vi "ANN on Simulated Starter Kit 1.0.vi"() -> ()   [LabVIEW 2017]
doc: "This VI demonstrates how to descontrol a simulated Starter Kit robot based on an Artificial Neural Network (ANN) algorithm. \n\nThe Starter Kit robot will track the path of red dots at the <b>Linear Velocity</b> you specify."
uses:
  ANN/ModelType.ctl
  ANN/ESN network/ESN_Network.ctl
  <vilib>/Analysis/Matrix/Datatypes/RealMatrix.ctl
  ANN/Trajectory.ctl
  <vilib>/robotics/Simulator/Engine/ctl/DeviceID.ctl
  <vilib>/Platform/TimedLoop/XDataNode/timing_clust.ctl
  <vilib>/Platform/TimedLoop/XDataNode/nitl_modes.ctl
  <vilib>/Platform/TimedLoop/XDataNode/wakeup.ctl
  ANN/ESN network/UserSettingsESN.ctl
  <vilib>/robotics/Simulator/Interface/Simulator References/Get Robot Body Reference.vi
  <vilib>/robotics/Simulator/Interface/Simulator References/Get World Reference.vi
  <instrlib>/DC Motor Controller/HAIOL/DC Motor Controller.lvclass
  <vilib>/Platform/TimedLoop/XDataNode/XDataNode.xnode
  <vilib>/robotics/Simulator/NI_Robotics_Simulator.lvlib
  <vilib>/Platform/TimedLoop/XDataNode/XDNodeRunTimeDep.lvlib
  <instrlib>/DC Motor Controller/HAIOL/Simulator/DC Motor Controller Simulator.lvclass
  <vilib>/Analysis/Matrix/NI_Matrix.lvlib
  <vilib>/gmath/NI_Gmath.lvlib
  <resource>/objmgr/LVODE.rc
panel:
  out "ESN trained 2":T1
  in  "Render Destination":enum16{"Scene Window", "Scene Display"}(ring)=enum."Scene Display"
  out "Location Error":cluster{"x":dbl, "y":dbl, "Orientation":dbl}(graph)
  out "Motor":dbl[][](graph)
  out "MSE":dbl
  in  "Linear Velocity":dbl=0.5 min=0.0 max=1.0 step=0.01
  in  "Model Type":T3=1 items=["Analytical Kinematic Model", "ANN Kinematic Model"]
  in  "Quit":bool
  out "Waveform WR_WL":dbl[][](graph)
  out "Time of Acquisition":i64
  out "Waveform V_W":dbl[][](graph)
  out "V_W":dbl[][](array[numeric])
  out "WR_WL":dbl[][](array[numeric])
  out "Data_WorkSpace":dbl[][](array[numeric])
  out "Percentage":string
  out "Data Acquisition Progress":dbl(slide) scale=0.0..100.0
  in  "WayPoints":cluster{sgl, sgl}[](array[cluster])=[{0.5, 0.5}, {0.5, 1.0}, {0.5, 1.5}, {0.5, 2.0}, {0.5, 2.5}, {0.5, 3.0}, {0.79999995, 3.4}, {1.2, 3.7}, {1.7, 3.7}, {2.1, 4.0}, {2.4, 4.4}, {2.7, 4.8}, {3.0, 5.2}, {3.4, 5.5}, {3.9, 5.5}, {4.4, 5.5}, {4.8, 5.8}, {5.3, 5.8}, {5.85, 5.5}, {5.85, 5.0}, {5.85, 4.5}, {5.4, 4.1}, {5.0, 3.8}, {4.7, 3.4}, {4.4, 3.0}, {4.1, 2.6}, {3.8, 2.2}, {3.8, 1.7}, {3.8, 1.2}, {4.1, 0.79999995}, {4.5, 0.5}, {5.0, 0.5}, {5.4, 0.79999995}]
  in  "method":i32(ring)=3 items=["nearest", "linear", "spline", "cubic Hermite"]
  in  "ntimes":i32=5
  out "trajectory":T4
  out "Path Graph":cluster{"yi":dbl[], "yi":dbl[]}[](graph)
  in  "Next":bool
  out "data acquisition status":bool
  in  "ESN trained":T1={"output to internal feedback?"=FALSE, "output to output feedback?"=FALSE, "input to output feedforward?"=TRUE, "number of input (K)"=2, "number of internal (N)"=222, "number of output (L)"=2, "input normalization vector"=[0.6006126900000001, 2.94100566], "output restore vector"=[30.199380389999998, 30.418265820000002], "input weight (N*K)"=array222x2[444 elements], "feedback weight (N*L)"=[], "internal weight (N*N)"=array222x222[49284 elements], "output weight (L*(K+N+L))"=array2x224[448 elements]}
  out "back status":bool
  out "3D Picture":refnum<vi>(3d-picture)
  # "Path Determintion"
  # "ANN Training"
  # "Mean\nSquare\nError"
  # "the range [0,1]."
  # "V,  W,  WL,  WR"
  # "Workspace Calculations"
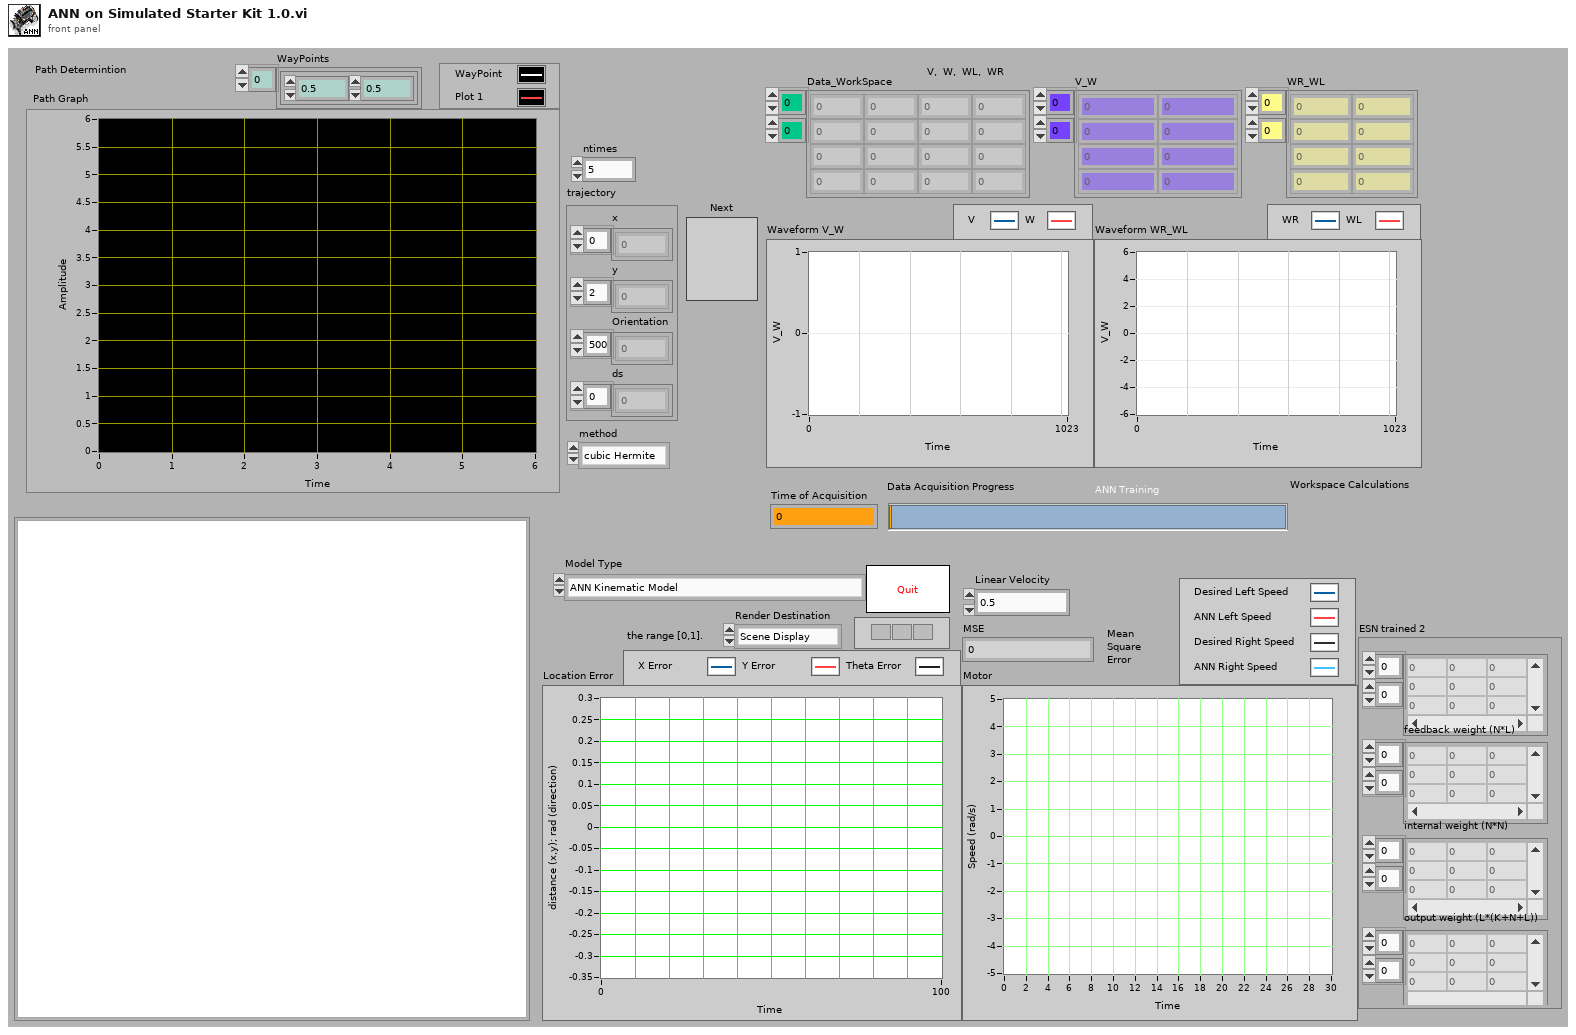
[diagram p1: front panel]
types:
  T1 = typedef "ESN_Network.ctl" = cluster{"output to internal feedback?":bool, "output to output feedback?":bool, "input to output feedforward?":bool, "number of input (K)":i32, "number of internal (N)":i32, "number of output (L)":i32, "input normalization vector":dbl[], "output restore vector":dbl[], "input weight (N*K)":T2, "feedback weight (N*L)":T2, "internal weight (N*N)":T2, "output weight (L*(K+N+L))":T2}
  T2 = typedef "NI_Matrix.lvlib/RealMatrix.ctl" = dbl[][]
  T3 = typedef "ModelType.ctl" = u16
  T4 = typedef "Trajectory.ctl" = cluster{"x":dbl[], "y":dbl[], "Orientation":dbl[], "ds":dbl[]}
  T5 = typedef "NI_Robotics_Simulator.lvlib/DeviceID.ctl" = cluster{"robot ID":string, "sensor/actuator ID":string}
  T6 = typedef "XDNodeRunTimeDep.lvlib/timing_clust.ctl" = cluster{"Expected End [f-1]":u64, "Actual End [f-1]":u64, "Finished Late? [f-1]":bool, "Expected End [i-1]":u64, "Actual End [i-1]":u64, "Finished Late? [i-1]":bool, "Expected Start [i]":u64, "Actual Start [i]":u64, "Expected Start [f]":u64, "Actual Start [f]":u64, "Source Name":string, "Structure Name":string, "Period":i64, "Deadline":i64, "Offset":i64, "Start":i64, "Priority":i32, "Timeout":i32, "Mode":T7, "Wakeup Reason":T8, "Error":errorcluster, "Source Type":string, "Secondary Source Type":string, "Global End Time":u64, "Global Start Time":u64, "Frame Duration":u64, "Iteration Duration":u64, "Assigned CPU":i32, "I/O Scan Engine Mode":u32}
  T7 = typedef "XDNodeRunTimeDep.lvlib/nitl_modes.ctl" = enum32{"No Change", "Process missed periods, maintain original phase", "Discard missed periods, maintain original phase", "Process missed periods, ignore original phase", "Discard missed periods, ignore original phase"}
  T8 = typedef "XDNodeRunTimeDep.lvlib/wakeup.ctl" = enum32{"Normal", "Aborted", "Asynchronous wakeup", "Timing source error", "Timed loop error", "Timeout"}
  T9 = typedef "UserSettingsESN.ctl" = cluster{"output to internal feedback?":bool, "output to output feedback?":bool, " input to output feedforward?":bool, "number of input (K)":i32, "number of internal (N)":i32, "number of output (L)":i32}
  T10 = typedef "VehiclePosture.ctl" = cluster{"x":dbl, "y":dbl, "Orientation":dbl}
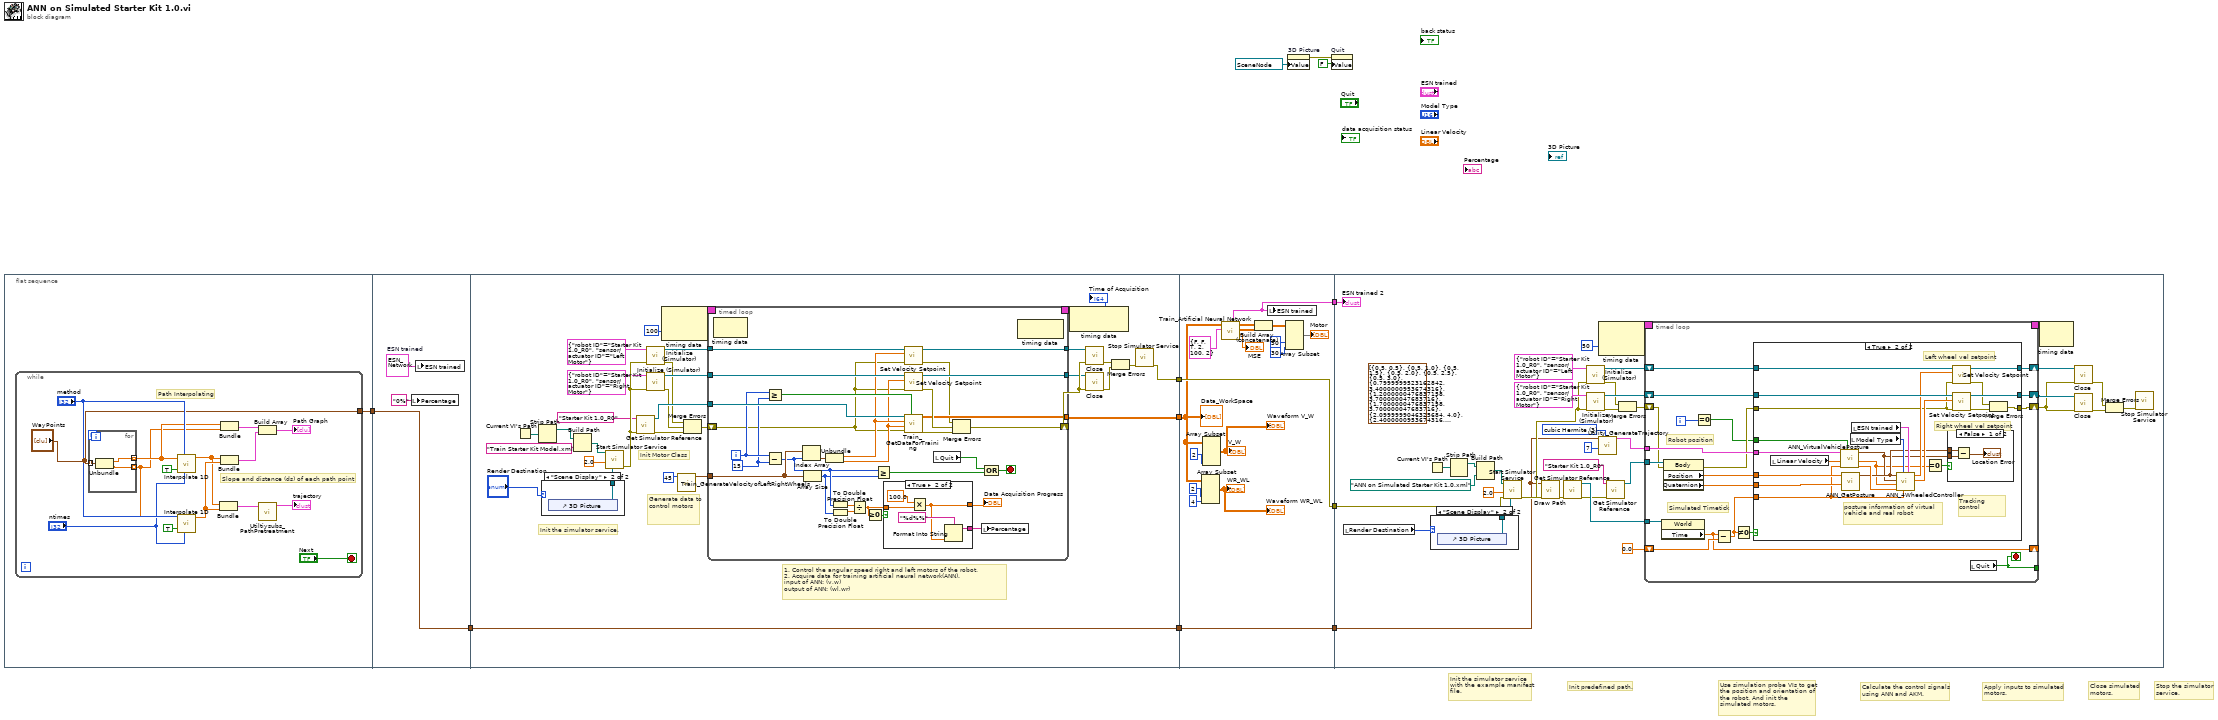
[diagram p0: block diagram]
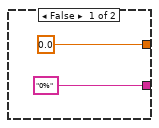
[diagram p2: hidden frame]
diagram:
  # "Init the simulator service\nwith the example manifest\nfile."
  # "Stop the simulator\nservice."
  # "Close simulated\nmotors."
  # "Apply inputs to simulated\nmotors."
  # "Calculate the control signals\nusing ANN and AKM."
  # "Use simulation probe VIs to get\nthe position and orientation of\nthe robot. And init the\nsimulated motors."
  # "Init predefined path."
  n1 = flat-sequence {
    tunnel: [w12] -> w6
    tunnel: w6 -> [w31]
    tunnel: [w31] -> w5
    tunnel: [w38] -> w7
    tunnel: w5 -> [w38]
    tunnel: [w37] -> w3
    tunnel: [w35] -> w2
    tunnel: [w119] -> w8
    tunnel: w7 -> [w119]
    tunnel: [w118] -> w4
    tunnel: w3 -> [w118]
    tunnel: w2 -> [w117]
    tunnel: [w111] -> w1
    tunnel: w8 -> [w130]
    tunnel: w4 -> [w131]
    tunnel: w1 -> [w128]
    frame #0 {
      n2 = while {
        tunnel: ["WayPoints"] -> w12
        stop <- "Next" stop-if-true
        # "Slope and distance (ds) of each path point"
        # "Path Interpolating"
        n3 = for {
          tunnel: "WayPoints" -> [w30] mode=indexing
          tunnel: [w29] -> w19 mode=indexing
          tunnel: [w28] -> w13 mode=indexing
          n4 = Unbundle(w30) -> (w29:sgl, w28:sgl)
        }
        n5 = call <vilib>:"Interpolate 1D.vi"("ntimes"="ntimes", "method"="method", "X is monotonic"=TRUE, "Y"=w19) -> ("yi"=w22:dbl[])  [unwired: 5 in, 2 out]
        n6 = call <vilib>:"Interpolate 1D.vi"("ntimes"="ntimes", "method"="method", "X is monotonic"=TRUE, "Y"=w13) -> ("yi"=w23:dbl[])  [unwired: 5 in, 2 out]
        n7 = Bundle("yi"=w22, "yi"=w23) -> (w24:cluster{"yi":dbl[], "yi":dbl[]})  [unwired: 1 in]
        n8 = Bundle("yi"=w22, "yi"=w23) -> (w20:cluster{"yi":dbl[], "yi":dbl[]})  [unwired: 1 in]
        n9 = Bundle(w19, w13) -> (w14:cluster{sgl[], sgl[]})  [unwired: 1 in]
        n10 = Build Array(w14, w20) -> (→"Path Graph":cluster{"yi":dbl[], "yi":dbl[]}[])
        n11 = call "Utiltiysubs_PathPretreatment.vi"("original trajectory"=w24) -> ("trajectory"=→"trajectory":T4)  [unwired: 10 in]
      }
    }
    frame #1 {
      w33 = T1 {"output to internal feedback?"=FALSE, "output to output feedback?"=FALSE, "input to output feedforward?"=TRUE, "number of input (K)"=2, "number of internal (N)"=222, "number of output (L)"=2, "input normalization vector"=[0.6006126900000001, 2.94100566], "output restore vector"=[30.199380389999998, 30.418265820000002], "input weight (N*K)"=array222x2[444 elements], "feedback weight (N*L)"=[], "internal weight (N*N)"=array222x222[49284 elements], "output weight (L*(K+N+L))"=array2x224[448 elements]}  # ESN trained
      n12 = local write "Percentage"("0%" ("Percentage")) -> ()
      n13 = local write "ESN trained"(w33) -> ()
    }
    frame #2 {
      # "1. Control the angular speed right and left motors of the robot.\n2. Acquire data for training artificial neural network(ANN).\ninput of ANN: (v,w)\noutput of ANN: (wl,wr)"
      # "Generate data to control motors"
      # "Init Motor Class"
      # "Init the simulator service."
      n14 = Current VI's Path() -> (path=w43:path)
      n15 = Strip Path(path=w43) -> (stripped path=w42:path)  [unwired: 1 out]
      n16 = case shown="\"Scene Display\"" "Render Destination" {
        tunnel: [_ w110] -> w40
        frame "Scene Window", Default {
        }
        frame "Scene Display" {
          n17 = control-ref of="3D Picture"() -> (w110:refnum<vi>)
        }
      }
      n18 = Build Path(base path=w42, name or relative path="Train Starter Kit Model.xml" ("ManifestFile")) -> (appended path=w41:path)
      n19 = call <vilib>:"Start Simulator Service.vi"("3D picture refnum"=w40, "step size (ms)"=2.0 ("stepsize(ms)"), "manifest file"=w41) -> ("error out"=w60:errorcluster)  [unwired: 8 in]
      n20 = call-poly <vilib>:"Get Simulator Reference.vi"("error in (no error)"=w60, "robot ID"="Starter Kit 1.0_R0") -> ("error out"=w45:errorcluster, "robot body ref"=w56:refnum<k20>)  [unwired: 8 in]
      n21 = call <instrlib>:"Initialize (Simulator).vi"("error in (no error)"=w60, "Device ID"=T5 {"robot ID"="Starter Kit 1.0_R0", "sensor/actuator ID"="Left Motor"}) -> ("error out"=w48:errorcluster, "DC Motor Controller out"=w53:refnum<class "DC Motor Controller.lvclass">)  [unwired: 8 in]
      n22 = call <instrlib>:"Initialize (Simulator).vi"("error in (no error)"=w60, "Device ID"=T5 {"robot ID"="Starter Kit 1.0_R0", "sensor/actuator ID"="Right Motor"}) -> ("error out"=w47:errorcluster, "DC Motor Controller out"=w54:refnum<class "DC Motor Controller.lvclass">)  [unwired: 8 in]
      n23 = node-c288(i64 100 ("Period")) -> (w66:T6)  [unwired: 1 in]
      n24 = call "Train_GenerateVelocityofLeftRightWheels.vi"("samples"=45) -> ("speed of Left and Right Wheels (rad/s)"=w55:cluster{dbl, dbl}[])  [unwired: 10 in]
      n25 = Merge Errors(w48, w47, w45) -> (w52:errorcluster)
      n26 = timed-loop {
        shift-right: [w95] -> w61
        shift-left: w52 -> [w72]
        tunnel: w53 -> [w94]
        tunnel: w54 -> [w93]
        tunnel: [w92] -> w58
        tunnel: [w91] -> w59
        tunnel: w55 -> [w90]
        tunnel: w56 -> [w88]
        tunnel: [w76] -> w35
        timing: w66 -> [_]
        timing-out: [_] -> w65
        i -> [w87]
        stop <- w74 stop-if-true
        w86 = 15 ("y")
        n27 = node-c288() -> ()  [unwired: 1 in, 1 out]
        n28 = Greater Or Equal?(x=w87, y=w86) -> (x >= y?=w85:bool)
        n29 = Subtract(x=w87, y=w86) -> (x-y=w89:i32)
        n30 = Index Array(array=w90, index=w89) -> (element=w84:cluster{dbl, dbl})
        n31 = Array Size(array=w90) -> (size(s)=w81:i32)
        n32 = Unbundle(w84) -> (w83:dbl, w82:dbl)
        n33 = To Double Precision Float(number=w89) -> (double precision float=w79:dbl)
        n34 = To Double Precision Float(number=w81) -> (double precision float=w80:dbl)
        n35 = Divide(x=w79, y=w80) -> (x/y=w70:dbl)
        n36 = Greater Or Equal To 0?(x=w70) -> (x >= 0?=w69:bool)
        n37 = Greater Or Equal?(x=w89, y=w81) -> (x >= y?=w75:bool)
        n38 = case shown="True" w69 {
          tunnel: w70 -> [_ w102]
          tunnel: ["0%" w99] -> w68
          tunnel: [0.0 w98] -> w67
          frame False {
          }
          frame True {
            n39 = Multiply(x=100.0 ("y"), y=w102) -> (x*y=w98:dbl)
            n40 = Format Into String(format string="%d%%", w98) -> (resulting string=w99:string)  [unwired: 2 in, 1 out]
          }
        }
        "Data Acquisition Progress" <- w67
        n41 = call-dynamic "Set Velocity Setpoint.vi"("error in (no error)"=w72, "CCW Velocity (0 rad/s)"=w83, "DC Motor Controller in"=w94) -> ("error out"=w71:errorcluster, "DC Motor Controller out"=w92:refnum<class "DC Motor Controller.lvclass">)  [unwired: 7 in]
        n42 = call-dynamic "Set Velocity Setpoint.vi"("error in (no error)"=w72, "CCW Velocity (0 rad/s)"=w82, "DC Motor Controller in"=w93) -> ("error out"=w77:errorcluster, "DC Motor Controller out"=w91:refnum<class "DC Motor Controller.lvclass">)  [unwired: 7 in]
        n43 = call "Train_GetDataForTraining.vi"("DataIn"=w85, "error in (no error)"=w72, "WR"=w82, "Wl"=w83, "robot body ref"=w88) -> ("error out"=w78:errorcluster, "Data"=w76:dbl[][])  [unwired: 5 in]
        n44 = local read "Quit"() -> (w73:bool)
        n45 = Merge Errors(w71, w77, w78) -> (w95:errorcluster)
        n46 = local write "Percentage"(w68) -> ()
        n47 = Compound Arithmetic op=OR(w73, w75) -> (w74:bool)
        n48 = node-c288() -> ()  [unwired: 1 in, 1 out]
      }
      n49 = node-c288(w65) -> (→"Time of Acquisition":i64)
      n50 = call-dynamic "Close.vi"("error in (no error)"=w61, "DC Motor Controller in"=w58) -> ("error out"=w62:errorcluster)  [unwired: 9 in]
      n51 = call-dynamic "Close.vi"("error in (no error)"=w61, "DC Motor Controller in"=w59) -> ("error out"=w63:errorcluster)  [unwired: 9 in]
      n52 = Merge Errors(w62, w63) -> (w64:errorcluster)
      n53 = call <vilib>:"Stop Simulator Service.vi"("error in (no error)"=w64) -> ("error out"=w37:errorcluster)  [unwired: 10 in]
    }
    frame #3 {
      n54 = Array Subset(array=w117, index (col)=2 ("index"), length (col)=4 ("length")) -> (→"WR_WL" →"Waveform WR_WL":dbl[][])  [unwired: 2 in]
      n55 = Array Subset(array=w117, length (col)=2 ("length")) -> (→"V_W" →"Waveform V_W":dbl[][])  [unwired: 3 in]
      n56 = call "Train_Artificial Neural Network.vi"("UserSettingsESN"=T9 {"output to internal feedback?"=FALSE, "output to output feedback?"=FALSE, " input to output feedforward?"=TRUE, "number of input (K)"=2, "number of internal (N)"=100, "number of output (L)"=2}, "Data"=w117) -> ("MSE"=→"MSE":dbl, "Wr"=w125:dbl[][], "Wl"=w126:dbl[][], "ESN trained"=w111:T1)  [unwired: 5 in, 1 out]
      n57 = Build Array (concatenate)(w126, w125) -> (w124:dbl[][])
      n58 = local write "ESN trained"(w111) -> ()
      n59 = Array Subset(array=w124, index (col)=50 ("index"), length (col)=30 ("length")) -> (→"Motor":dbl[][])  [unwired: 2 in]
      "Data_WorkSpace" <- w117
    }
    frame #4 {
      (unwired) cluster{sgl, sgl}[] [{0.5, 0.5}, {0.5, 1.0}, {0.5, 1.5}, {0.5, 2.0}, {0.5, 2.5}, {0.5, 3.0}, {0.79999995, 3.4}, {1.2, 3.7}, {1.7, 3.7}, {2.1, 4.0}, {2.4, 4.4}, {2.7, 4.8}, {3.0, 5.2}, {3.4, 5.5}, {3.9, 5.5}, {4.4, 5.5}, {4.8, 5.8}, {5.3, 5.8}, {5.85, 5.5}, {5.85, 5.0}, {5.85, 4.5}, {5.4, 4.1}, {5.0, 3.8}, {4.7, 3.4}, {4.4, 3.0}, {4.1, 2.6}, {3.8, 2.2}, {3.8, 1.7}, {3.8, 1.2}, {4.1, 0.79999995}, {4.5, 0.5}, {5.0, 0.5}, {5.4, 0.79999995}] ("WayPoints")
      w160 = 3 items=["nearest", "linear", "spline", "cubic Hermite", "Lagrange"] ("method")
      n60 = local read "Render Destination"() -> (w129:enum16{"Scene Window", "Scene Display"})
      n61 = Current VI's Path() -> (path=w157:path)
      n62 = case shown="\"Scene Display\"" w129 {
        tunnel: [_ w165] -> w147
        frame "Scene Window", Default {
        }
        frame "Scene Display" {
          n63 = control-ref of="3D Picture"() -> (w165:refnum<vi>)
        }
      }
      n64 = Strip Path(path=w157) -> (stripped path=w156:path)  [unwired: 1 out]
      n65 = Build Path(base path=w156, name or relative path=path "ANN on Simulated Starter Kit 1.0.xml" ("Simulation Manifest File")) -> (appended path=w155:path)
      n66 = call <vilib>:"Start Simulator Service.vi"("3D picture refnum"=w147, "error in (no error)"=w131, "step size (ms)"=2.0 ("stepsize(ms)"), "manifest file"=w155) -> ("error out"=w159:errorcluster)  [unwired: 7 in]
      n67 = call "Draw Path.vi"("error in (no error)"=w159, "WayPoints"=w130) -> ("error out"=w141:errorcluster)  [unwired: 9 in]
      n68 = call-poly <vilib>:"Get Simulator Reference.vi"("error in (no error)"=w141) -> ("error out"=w140:errorcluster, "world ref"=w142:refnum<k20>)  [unwired: 9 in]
      n69 = node-c288(i64 50) -> (w164:T6)  [unwired: 1 in]
      n70 = call "Utility_GenerateTrajectory.vi"("method"=w160, "ntimes"=7, "path"=w130) -> ("trajectory"=w162:T4)  [unwired: 8 in]
      n71 = call-poly <vilib>:"Get Simulator Reference.vi"("error in (no error)"=w140, "robot ID"="Starter Kit 1.0_R0" ("Robot ID")) -> ("error out"=w132:errorcluster, "robot body ref"=w143:refnum<k20>)  [unwired: 8 in]
      n72 = call <instrlib>:"Initialize (Simulator).vi"("error in (no error)"=w132, "Device ID"=T5 {"robot ID"="Starter Kit 1.0_R0", "sensor/actuator ID"="Left Motor"}) -> ("error out"=w137:errorcluster, "DC Motor Controller out"=w146:refnum<class "DC Motor Controller.lvclass">)  [unwired: 8 in]
      n73 = call <instrlib>:"Initialize (Simulator).vi"("error in (no error)"=w132, "Device ID"=T5 {"robot ID"="Starter Kit 1.0_R0", "sensor/actuator ID"="Right Motor"}) -> ("error out"=w139:errorcluster, "DC Motor Controller out"=w149:refnum<class "DC Motor Controller.lvclass">)  [unwired: 8 in]
      n74 = Merge Errors(w137, w139) -> (w138:errorcluster)
      n75 = timed-loop {
        shift-right: [w175] -> w136
        shift-left: w138 -> [w169]
        tunnel: w143 -> [w184]
        tunnel: w162 -> [w181]
        timing: w164 -> [_]
        timing-out: [_] -> w163
        shift-right: [w180] -> w154
        shift-left: w146 -> [w183]
        shift-right: [w179] -> w153
        shift-left: w149 -> [w182]
        tunnel: w142 -> [w174]
        shift-right: [w172] -> _
        shift-left: 0.0 ("y") -> [w173]
        tunnel: [w166] -> _
        i -> [w168]
        stop <- w166 stop-if-true
        # "Simulated Timetick"
        # "Robot position"
        n76 = property class="World"(reference=w174) -> ("Time"=w172:sgl)  [unwired: 1 in, 2 out]
        n77 = property class="Body"(reference=w184, error in=w169) -> (error out=w176:errorcluster, "Position"=w178:sgl[], "Quaternion"=w177:sgl[])  [unwired: 1 out]
        n78 = Equal To 0?(x=w168) -> (x = 0?=w167:bool)
        n79 = Subtract(x=w172, y=w173) -> (x-y=w170:dbl)
        n80 = Not Equal To 0?(x=w170) -> (x != 0?=w171:bool)
        n81 = case shown="True" w171 {
          tunnel: w183 -> [w187 w210]
          tunnel: w182 -> [w186 w209]
          tunnel: w181 -> [_ w208]
          tunnel: [w187 w207] -> w180
          tunnel: [w186 w206] -> w179
          tunnel: w178 -> [_ w205]
          tunnel: w177 -> [_ w204]
          tunnel: w176 -> [w185 w199]
          tunnel: [w185 w196] -> w175
          tunnel: w170 -> [_ w200]
          tunnel: w167 -> [_ w190]
          frame False {
          }
          frame True {
            # "Tracking control"
            # "posture information of virtual vehicle and real robot"
            # "Right wheel vel setpoint"
            # "Left wheel vel setpoint"
            n82 = local read "Linear Velocity"() -> (w193:dbl)
            n83 = call "ANN_VirtualVehiclePosture.vi"("reset"=w190, "dt"=w200, "linear velocity"=w193, "trajectory"=w208) -> ("angular velocity"=w201:dbl, "velocity"=w189:dbl, "virtual posture"=w191:T10)  [unwired: 5 in]
            n84 = call "ANN_GetPosture.vi"("quaternion"=w204, "position"=w205) -> ("vehicle status"=w192:T10)  [unwired: 9 in]
            n85 = local read "Model Type"() -> (w194:T3)
            n86 = local read "ESN trained"() -> (w195:T1)
            n87 = call "ANN_4WheeledController.vi"("ESN trained"=w195, "dt"=w200, "model type"=w194, "wref (nan)"=w201, "vref (nan)"=w189, "desired posture"=w191, "current posture"=w192) -> ("wr"=w202:dbl, "wl"=w203:dbl)  [unwired: 3 in]
            n88 = Equal To 0?(x=w189) -> (x = 0?=w188:bool)
            n89 = case shown="False" w188 {
              tunnel: w192 -> [w213 _]
              tunnel: w191 -> [w212 _]
              frame False {
                n90 = Subtract(x=w213, y=w212) -> (x-y=→"Location Error":T10)
              }
              frame True {
              }
            }
            n91 = call-dynamic "Set Velocity Setpoint.vi"("error in (no error)"=w199, "CCW Velocity (0 rad/s)"=w203, "DC Motor Controller in"=w210) -> ("error out"=w197:errorcluster, "DC Motor Controller out"=w207:refnum<class "DC Motor Controller.lvclass">)  [unwired: 7 in]
            n92 = call-dynamic "Set Velocity Setpoint.vi"("error in (no error)"=w199, "CCW Velocity (0 rad/s)"=w202, "DC Motor Controller in"=w209) -> ("error out"=w198:errorcluster, "DC Motor Controller out"=w206:refnum<class "DC Motor Controller.lvclass">)  [unwired: 7 in]
            n93 = Merge Errors(w197, w198) -> (w196:errorcluster)
          }
        }
        n94 = local read "Quit"() -> (w166:bool)
      }
      n95 = node-c288(w163) -> ()  [unwired: 1 out]
      n96 = call-dynamic "Close.vi"("error in (no error)"=w136, "DC Motor Controller in"=w154) -> ("error out"=w134:errorcluster)  [unwired: 9 in]
      n97 = call-dynamic "Close.vi"("error in (no error)"=w136, "DC Motor Controller in"=w153) -> ("error out"=w135:errorcluster)  [unwired: 9 in]
      n98 = Merge Errors(w134, w135) -> (w133:errorcluster)
      n99 = call <vilib>:"Stop Simulator Service.vi"("error in (no error)"=w133) -> ()  [unwired: 10 in, 1 out]
      "ESN trained 2" <- w128
    }
  }
  n100 = property on="3D Picture" class="SceneGraphDisp (strict)"("Value"=refnum<vi> refnum ("3D Picture")) -> (error out=w10:errorcluster)  [unwired: 2 in, 1 out]
  n101 = property on="Quit" class="Bool (strict)"(error in=w10, "Value"=FALSE ("Quit")) -> ()  [unwired: 1 in, 2 out]
